vi "Replace Space With Comma.vi"(8 "error in (no error)":errorcluster, 10 "Input":string, 11 "Tovey 9150 in":refnum<class "Tovey 9150.lvclass">) -> (0 "error out":errorcluster, 2 "Output":string, 3 "Tovey 9150 out":refnum<class "Tovey 9150.lvclass">)   [LabVIEW 2015, in "Tovey 9150.lvclass"]
uses:
  Tovey 9150.lvclass
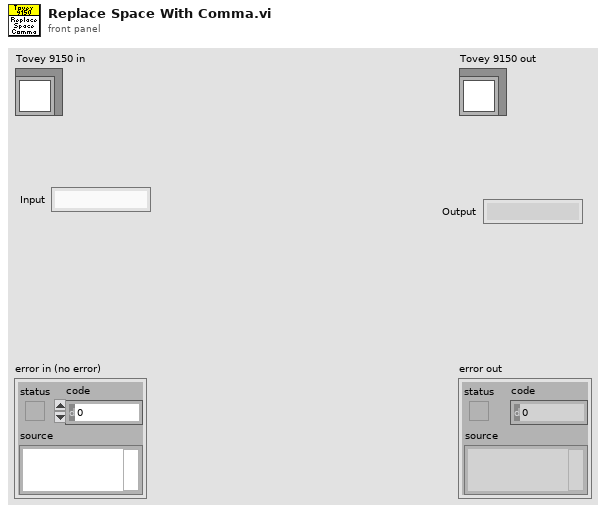
[diagram p1: front panel]
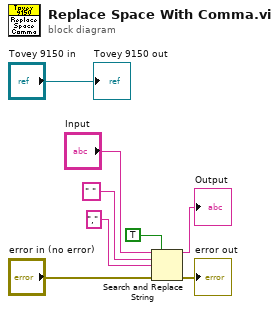
[diagram p0: block diagram]
diagram:
  n1 = Search and Replace String(replace all?=TRUE ("replace all? (F)"), input string="Input", search string=" ", replace string="," ("substring (\"\")"), error in="error in (no error)") -> (result string=→"Output":string, error out=→"error out":errorcluster)  [unwired: 3 in, 2 out]
  "Tovey 9150 out" <- "Tovey 9150 in"
